vi "TCP-IP Mgr.Read-Write.vi"(6 "Rcv Q.Element":T1={"Cmd"="Task", "Sub"="TCP-IP Rcv", "Data1"=variant, "Data2"=variant}, 7 "Q Local":refnum<queue>, 8 "error in":errorcluster, 9 "Q.Rcv":refnum<queue>, 10 "Q Send":refnum<queue>, 11 "TCPIP ID":refnum<k5>) -> (0 "error out":errorcluster, 2 "Disconnect/Exit":bool)   [LabVIEW 2024, in "EQMF.lvlib" / "TCP-IP.lvlib"]
uses:
  TCP-IP.lvlib
  Queues/Q.Element.ctl
  Queues/Queue Utils.lvlib
panel:
  out "Read Closed":bool
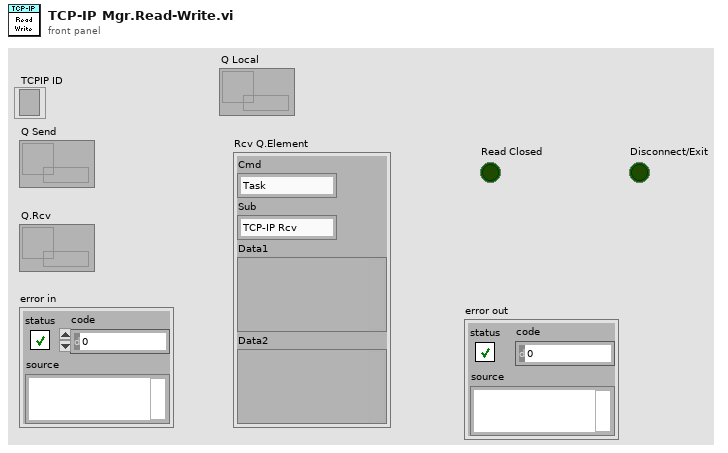
[diagram p1: front panel]
types:
  T1 = typedef "EQMF.lvlib/Queue Utils.lvlib/Q.Element.ctl" = cluster{"Cmd":string, "Sub":string, "Data1":variant, "Data2":variant}
  T2 = enum16{"Standard", "Buffered", "CRLF", "Immediate"}
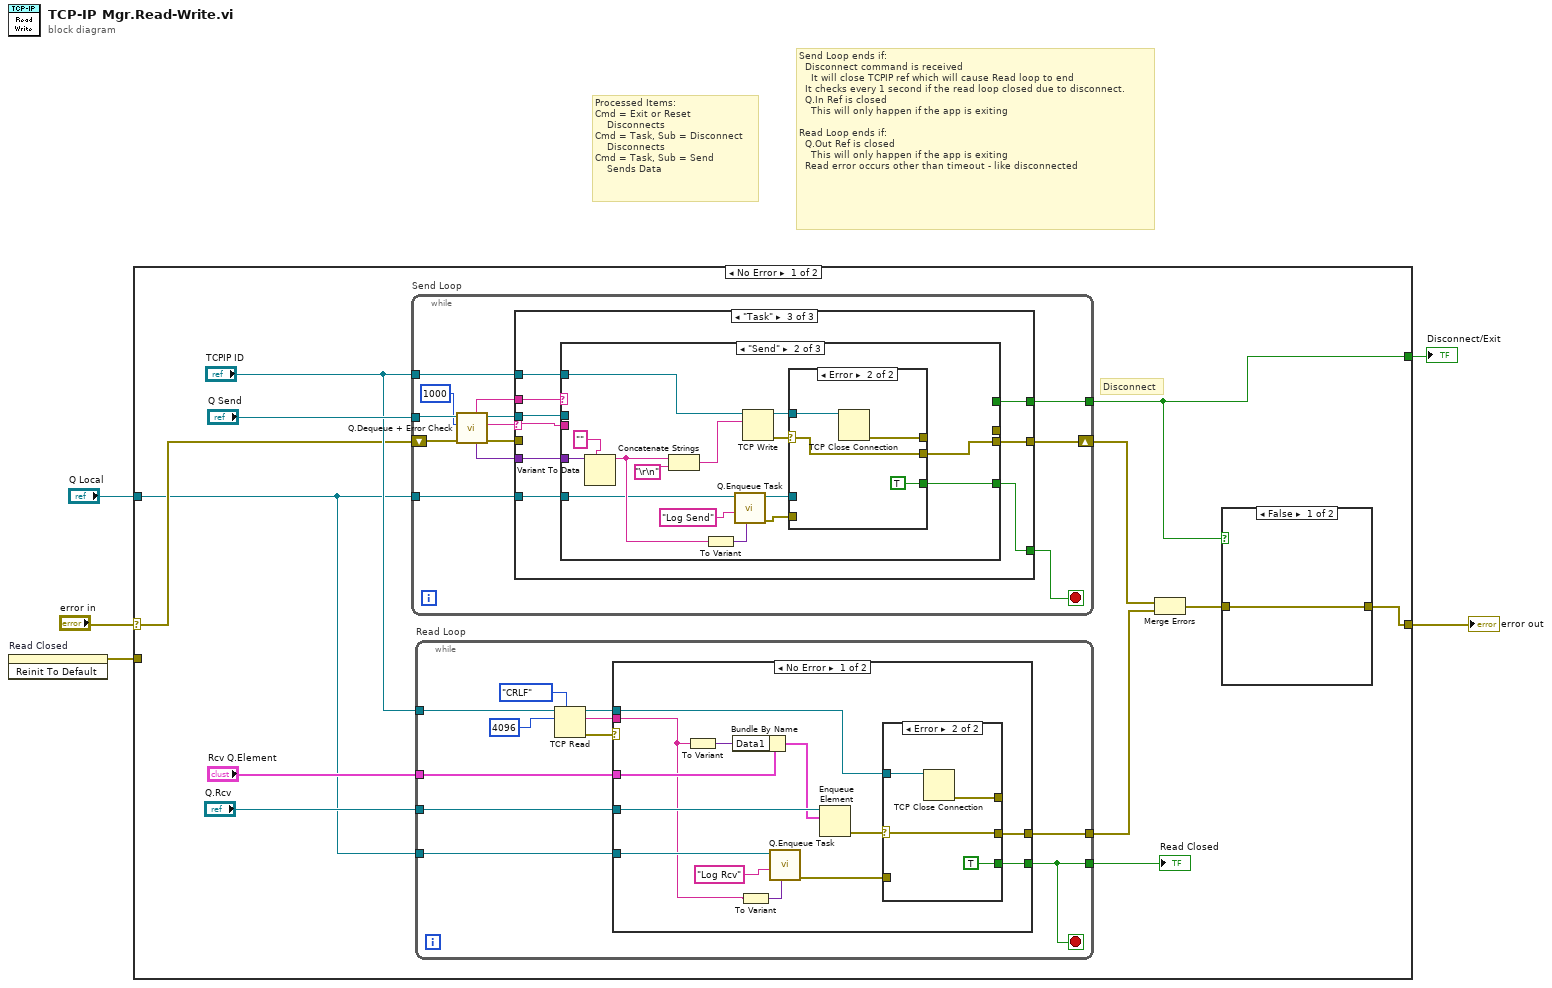
[diagram p0: block diagram]
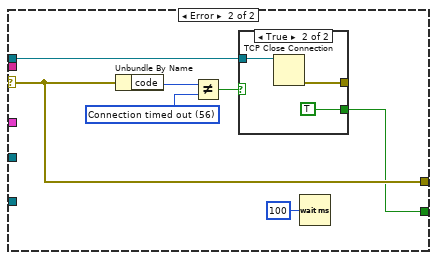
[diagram p4: hidden frame]
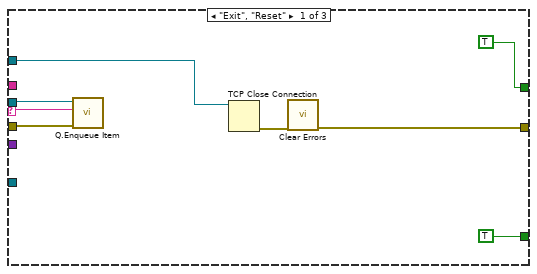
[diagram p6: hidden frame]
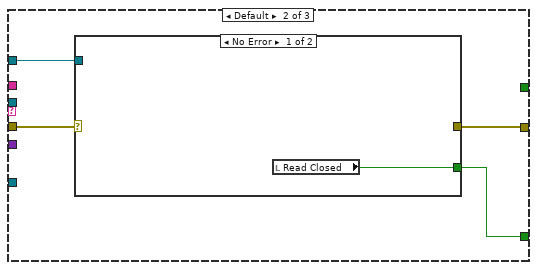
[diagram p7: hidden frame]
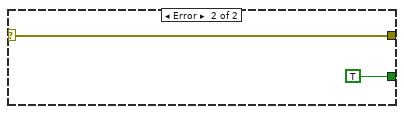
[diagram p8: hidden frame]
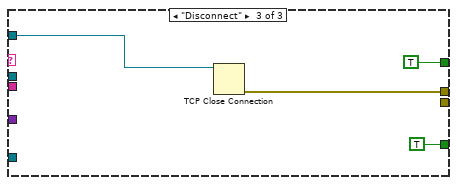
[diagram p11: hidden frame]
diagram:
  # "Send Loop ends if:\n  Disconnect command is received\n    It will close TCPIP ref which will cause Read loop to end\n  It checks every 1 second if the read loop closed due to disconnect.\n  Q.In Ref is closed\n    This will only happen if the app is exiting\n\nRead Loop ends if:\n  Q.Out Ref is closed\n    This will only happen if the app is exiting\n  Read error occurs other than timeout - like disconnected"
  # "Processed Items:\nCmd = Exit or Reset\n    Disconnects\nCmd = Task, Sub = Disconnect\n    Disconnects\nCmd = Task, Sub = Send\n    Sends Data"
  n1 = invoke on="Read Closed" class="Bool (strict)" method="Reinit To Default"() -> (error out=w3:errorcluster)  [unwired: 3 in, 2 out]
  n2 = case shown="No Error" "error in" {
    selector: "error in" -> [w14 w117]
    tunnel: [w9 w117] -> w5
    tunnel: w3 -> [_ _]
    tunnel: "Q Local" -> [w7 _]
    tunnel: [w6 _] -> w1
    frame No Error {
      # "Disconnect"
      n3 = while "Send Loop" {
        tunnel: "Q Send" -> [w69]
        tunnel: "TCPIP ID" -> [w67]
        shift-right: [w63] -> w12
        shift-left: w14 -> [w64]
        tunnel: [w59] -> w6
        tunnel: w7 -> [w57]
        stop <- w62 stop-if-true
        n4 = call "Q.Dequeue + Error Check.vi"("Error In"=w64, "Timeout(-1)"=1000, "Q In"=w69) -> ("error out"=w65:errorcluster, "Cmd"=w68:string, "Q Out"=w66:refnum<queue>, "Data1"=w60:variant, "Sub"=w61:string)  [unwired: 3 in, 1 out]
        n5 = case shown="\"Task\"" w68 {
          selector: w68 -> [w75 _ w89]
          tunnel: w67 -> [w77 w79 w91]
          tunnel: w66 -> [w76 _ w90]
          tunnel: w65 -> [w74 w81 _]
          tunnel: [w72 w78 w88] -> w63
          tunnel: [TRUE w80 w87] -> w62
          tunnel: w61 -> [_ _ w93]
          tunnel: w60 -> [_ _ w92]
          tunnel: [TRUE _ w86] -> w59
          tunnel: w57 -> [_ _ w85]
          frame "Exit", "Reset" {
            n6 = call "Q.Enqueue Item.vi"("Error In"=w74, "Cmd"=w75, "Q In"=w76) -> ()  [unwired: 7 in, 2 out]
            n7 = TCP Close Connection(connection ID=w77) -> (error out=w73:errorcluster)  [unwired: 2 in, 1 out]
            n8 = call <vilib>:"Clear Errors.vi"("error in (no error)"=w73) -> ("error out"=w72:errorcluster)  [unwired: 5 in, 1 out]
          }
          frame Default {
            n9 = case shown="No Error" w81 {
              selector: w81 -> [_ w83]
              tunnel: [w82 TRUE] -> w80
              tunnel: w79 -> [_ _]
              tunnel: [_ w83] -> w78
              frame No Error {
                n10 = local read "Read Closed"() -> (w82:bool)
              }
              frame Error {
              }
            }
          }
          frame "Task" {
            n11 = case shown="\"Send\"" w93 {
              tunnel: w92 -> [_ w107 _]
              tunnel: w91 -> [_ w104 w116]
              tunnel: w90 -> [_ _ _]
              tunnel: w89 -> [_ _ _]
              tunnel: [_ w101 _] -> w88
              tunnel: [_ w100 TRUE] -> w87
              tunnel: [_ _ TRUE] -> w86
              tunnel: [_ _ w113] -> _
              tunnel: w85 -> [_ w96 _]
              frame Default {
                # "Ignore other tasks.\nShould not receive any"
              }
              frame "Send" {
                n12 = Variant To Data(type="", Variant=w107) -> (data=w97:string)  [unwired: 1 in, 1 out]
                n13 = Concatenate Strings(w97, "\r\n") -> (w105:string)
                n14 = To Variant(anything=w97) -> (Variant=w98:variant)
                n15 = call "Q.Enqueue Task.vi"("Data1"=w98, "Task Name"="Log Send", "Q In"=w96) -> ("error out"=w94:errorcluster, "Q Out"=w95:refnum<queue>)  [unwired: 7 in]
                n16 = TCP Write(connection ID=w104, data in=w105) -> (connection ID out=w102:refnum<k5>, error out=w103:errorcluster)  [unwired: 2 in, 1 out]
                n17 = case shown="Error" w103 {
                  selector: w103 -> [_ w111]
                  tunnel: w102 -> [_ w112]
                  tunnel: [_ w111] -> w101
                  tunnel: [_ TRUE] -> w100
                  tunnel: [_ w109] -> _
                  tunnel: w95 -> [_ _]
                  tunnel: w94 -> [_ _]
                  frame No Error {
                  }
                  frame Error {
                    n18 = TCP Close Connection(connection ID=w112) -> (error out=w109:errorcluster)  [unwired: 2 in, 1 out]
                  }
                }
              }
              frame "Disconnect" {
                n19 = TCP Close Connection(connection ID=w116) -> (error out=w113:errorcluster)  [unwired: 2 in, 1 out]
              }
            }
          }
        }
      }
      n20 = while "Read Loop" {
        tunnel: "TCPIP ID" -> [w28]
        tunnel: "Q.Rcv" -> [w25]
        tunnel: "Rcv Q.Element" -> [w23]
        tunnel: [w21] -> w11
        tunnel: [w20] -> w8
        tunnel: w7 -> [w19]
        stop <- w20 stop-if-true
        n21 = TCP Read(connection ID=w28, bytes to read=4096, 7:T2."CRLF" ("mode (standard)")) -> (connection ID out=w22:refnum<k5>, data out=w26:string, error out=w24:errorcluster)  [unwired: 2 in]
        n22 = case shown="No Error" w24 {
          selector: w24 -> [_ w48]
          tunnel: w26 -> [w30 _]
          tunnel: w25 -> [w42 _]
          tunnel: w23 -> [w40 _]
          tunnel: [w36 w48] -> w21
          tunnel: w22 -> [w37 w51]
          tunnel: [w35 w47] -> w20
          tunnel: w19 -> [w32 _]
          frame No Error {
            n23 = To Variant(anything=w30) -> (Variant=w39:variant)
            n24 = Bundle By Name(cluster=w40, "Data1"=w39) -> (w41:T1)
            n25 = To Variant(anything=w30) -> (Variant=w34:variant)
            n26 = call "Q.Enqueue Task.vi"("Data1"=w34, "Task Name"="Log Rcv", "Q In"=w32) -> ("error out"=w31:errorcluster)  [unwired: 7 in, 1 out]
            n27 = Enqueue Element(queue=w42, element=w41) -> (error out=w38:errorcluster)  [unwired: 2 in, 2 out]
            n28 = case shown="Error" w38 {
              selector: w38 -> [_ w44]
              tunnel: w37 -> [_ w46]
              tunnel: [_ w44] -> w36
              tunnel: [_ TRUE] -> w35
              tunnel: [_ w43] -> _
              tunnel: w31 -> [_ _]
              frame No Error {
              }
              frame Error {
                n29 = TCP Close Connection(connection ID=w46) -> (error out=w43:errorcluster)  [unwired: 2 in, 1 out]
              }
            }
          }
          frame Error {
            w53 = 56 items=["No Error", "Argument Error", "Memory Full", "Out of Zone", "End of File", "File Already Open", "Generic File IO Error", "File Not Found", "File Permission Error", "Disk Full", "Duplicate Path", "Too Many Files Open", "Not Enabled", "Resource File Not Found", "Cannot Add Resource", "Resource Not Found", "Image Not Found", "Image Memory Error", "Pen Does Not Exist", "Config Bad Type", "Config Token Not Found", "Config Parse Error", "Config Memory Error", "Bad External Code Format", "Bad External Code Offset", "External Code Not Present", "Null Window", "Destroy Window Mixup", "Null Menu", "Print Aborted", "Bad Print Record", "Print Driver Error", "Windows Error During Print", "Memory Error During Print", "Print Dialog Error", "Generic Print Error", "Invalid Device Refnum", "Device Not Found", "Device Parameter Error", "Device Unit Error", "Can't Open Device", "Device Call Aborted", "Generic Error", "Cancelled By User", "Object ID Too Low", "Object ID Too High", "Object Not In Heap", "Unknown Heap", "Bad DefProc ID", "DefProc Not In Table", "Message Out Of Range", "Null Method", "Unknown Message", "Manager Call Not Supported", "Bad address", "Connection In progress", "Connection timed out", "Connection is already in progress", "Network attribute not supported", "Network error", "Address in use", "System out of memory", "Connection aborted", "Connection refused", "Connection is not connected", "Connection is already connected", "Connection closed", "Initialize error (interapplication manager)", "Bad occurrence", "Wait on unbound occurrence handler", "Occurrence queue overflow", "Bad path", "Semaphore not signaled", "Unrecognized type (interapplication manager)"] ("2nd Error to Convert")
            n30 = Unbundle By Name(w48) -> ("code"=w52:i32)
            n31 = Not Equal?(x=w52, y=w53) -> (x != y?=w50:bool)
            n32 = case shown="True" w50 {
              tunnel: w51 -> [_ w56]
              tunnel: [_ TRUE] -> w47
              tunnel: [_ w54] -> _
              frame False {
              }
              frame True {
                n33 = TCP Close Connection(connection ID=w56) -> (error out=w54:errorcluster)  [unwired: 2 in, 1 out]
              }
            }
            n34 = Wait (ms)(milliseconds to wait=u32 100) -> ()  [unwired: 1 out]
          }
        }
      }
      "Read Closed" <- w8
      n35 = Merge Errors(w12, w11) -> (w10:errorcluster)
      n36 = case shown="False" w6 {
        tunnel: w10 -> [w18 _]
        tunnel: [w18 _] -> w9
        frame False {
        }
        frame True {
        }
      }
    }
    frame Error {
    }
  }
  "error out" <- w5
  "Disconnect/Exit" <- w1
